vi "Set Run Ref.vi"(8 "error in (no error)":errorcluster, 10 "Run Ref":refnum<k24>, 11 "xwpfRun in":refnum<class "xwpfRun.lvclass">) -> (0 "error out":errorcluster, 3 "xwpfRun out":refnum<class "xwpfRun.lvclass">)   [LabVIEW 2017, in "Word_Specific.lvlib" / "xwpfRun.lvclass"]
uses:
  xwpfRun.lvclass
  C:/Users/Neo/Desktop/Dev_Tools_BR/LabVIEW_NPOI/lib/NPOI 2.1.1/NPOI.OOXML.dll
  lib/NPOI 2.1.1/NPOI.OOXML.dll
  xwpfRun.lvclass/xwpfRun.ctl
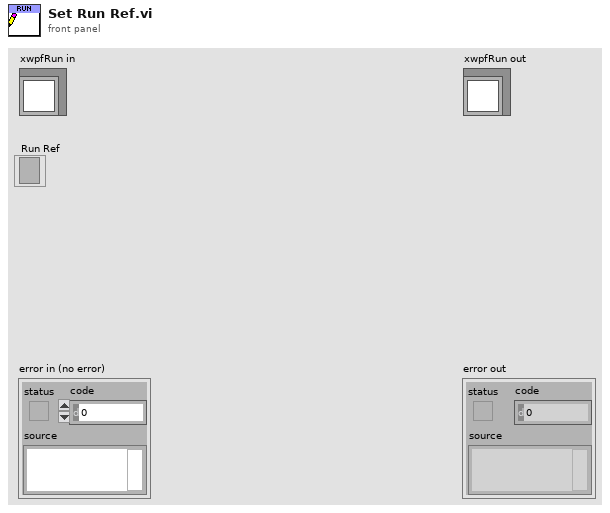
[diagram p1: front panel]
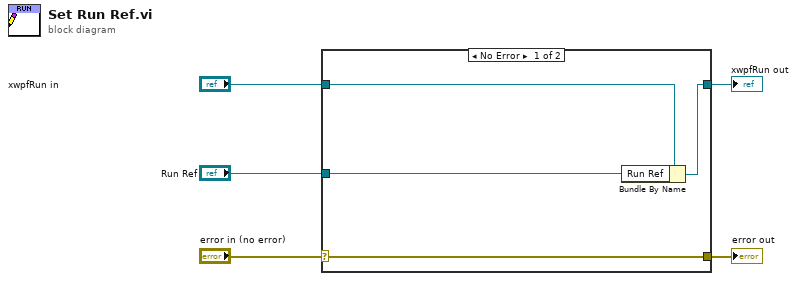
[diagram p0: block diagram]
diagram:
  n1 = case shown="No Error" "error in (no error)" {
    selector: "error in (no error)" -> [w9 w10]
    tunnel: [w9 w10] -> w4
    tunnel: [w7 w11] -> w2
    tunnel: "xwpfRun in" -> [w8 w11]
    tunnel: "Run Ref" -> [w6 _]
    frame No Error {
      n2 = Bundle By Name(cluster=w8, "Run Ref"=w6) -> (w7:refnum<class "xwpfRun.lvclass">)
    }
    frame Error {
    }
  }
  "error out" <- w4
  "xwpfRun out" <- w2
